vi "WSVCAP SHL Host LL I2C Build Socket Mask.vi"(0 "DUT Mask Array":bool[][](array[boolean]), 7 "DUT Mask Mode (Custom)":T1) -> (4 "Socket Mask Set [U64]":u64[](array[numeric]) format="%012x")   [LabVIEW 2012]
uses:
  Type Defs/WSVCAP SHL I2C DUT Mask Mode Enum.ctl
panel:
  # "DUT 01"
  # "DUT 02"
  # "DUT 03"
  # "DUT 04"
  # "DUT 05"
  # "DUT 06"
  # "DUT 07"
  # "DUT 08"
  # "DUT 09"
  # "DUT 10"
  # "DUT 11"
  # "DUT 12"
  # "DUT 13"
  # "DUT 14"
  # "DUT 15"
  # "DUT 16"
  # "DUT 17"
  # "DUT 18"
  # "DUT 19"
  # "DUT 20"
  # "DUT 21"
  # "DUT 22"
  # "DUT 23"
  # "DUT 24"
  # "DUT 25"
  # "DUT 26"
  # "DUT 27"
  # "DUT 28"
  # "DUT 29"
  # "DUT 30"
  # "DUT 31"
  # "DUT 32"
  # "DUT 33"
  # "DUT 34"
  # "DUT 35"
  # "DUT 36"
  # "C1"
  # "C2"
  # "C3"
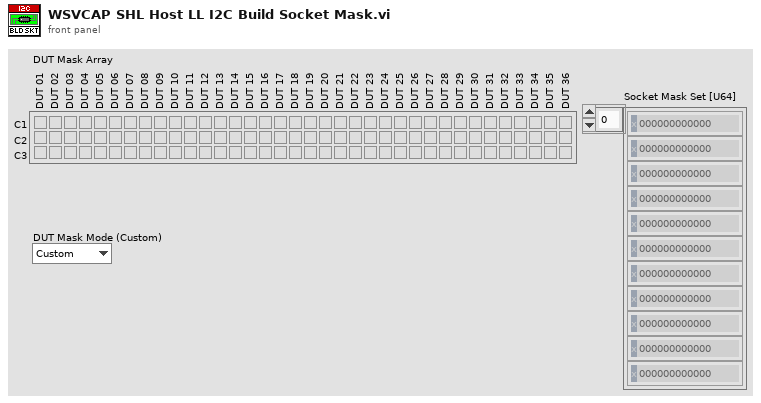
[diagram p1: front panel]
types:
  T1 = typedef "WSVCAP SHL I2C DUT Mask Mode Enum.ctl" = enum16{"Custom", "C1", "C2", "C3", "All"}
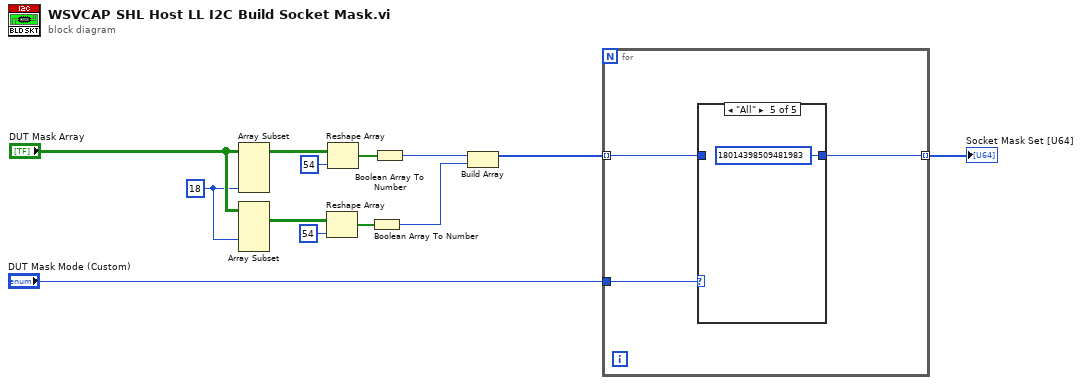
[diagram p0: block diagram]
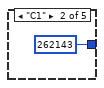
[diagram p3: hidden frame]
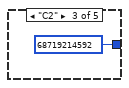
[diagram p4: hidden frame]
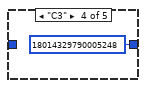
[diagram p5: hidden frame]
diagram:
  w11 = 18 ("index")
  n1 = Array Subset(array="DUT Mask Array", length (col)=w11) -> (w10:bool[][])  [unwired: 3 in]
  n2 = Array Subset(array="DUT Mask Array", index (col)=w11) -> (w7:bool[][])  [unwired: 3 in]
  n3 = Reshape Array(w7, 54 ("dimension size")) -> (w5:bool[])
  n4 = Reshape Array(w10, 54 ("dimension size")) -> (w6:bool[])
  n5 = Boolean Array To Number(Boolean array=w5) -> (number=w4:u64)
  n6 = Boolean Array To Number(Boolean array=w6) -> (number=w3:u64)
  n7 = Build Array(w3, w4) -> (w2:u64[])
  n8 = for {
    tunnel: "DUT Mask Mode (Custom)" -> [w16]
    tunnel: w2 -> [w15] mode=indexing
    tunnel: [w14] -> w1 mode=indexing
    n9 = case shown="\"All\"" w16 {
      tunnel: [w17 u64 262143 ("Socket Mask [U64]") u64 68719214592 ("Socket Mask [U64]") u64 18014329790005248 ("Socket Mask [U64]") u64 18014398509481983 ("Socket Mask [U64]")] -> w14
      tunnel: w15 -> [w17 _ _ _ _]
      frame "Custom" {
      }
      frame "C1" {
      }
      frame "C2" {
      }
      frame "C3" {
      }
      frame "All" {
      }
    }
  }
  "Socket Mask Set [U64]" <- w1
